vi "OrientationStateMachine.vi"(8 "Rubik's Moves":T1, 11 "Initial Orientation":T2) -> (3 "Final Orientation":T2)   [LabVIEW 2017]
uses:
  Controls/OrientationState.ctl
  Controls/RubikMoves.ctl
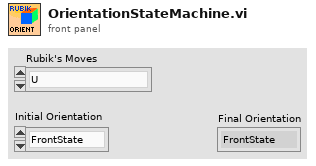
[diagram p1: front panel]
types:
  T1 = typedef "RubikMoves.ctl" = enum16{"U", "U'", "F", "F'", "D", "D'", "B", "B'", "L", "L'", "R", "R'"}
  T2 = typedef "OrientationState.ctl" = enum16{"FrontState", "UpState", "BackState", "DownState"}
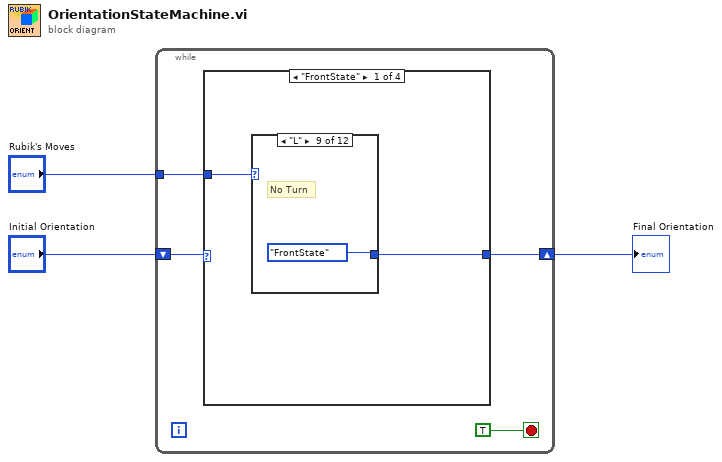
[diagram p0: block diagram]
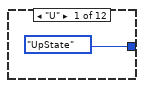
[diagram p2: hidden frame]
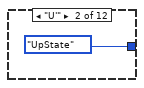
[diagram p3: hidden frame]
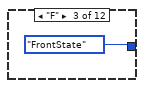
[diagram p4: hidden frame]
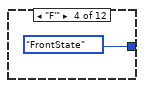
[diagram p5: hidden frame]
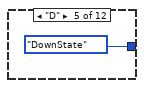
[diagram p6: hidden frame]
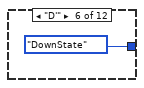
[diagram p7: hidden frame]
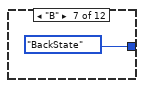
[diagram p8: hidden frame]
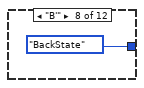
[diagram p9: hidden frame]
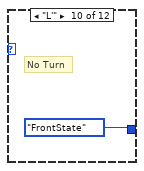
[diagram p10: hidden frame]
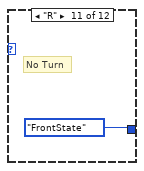
[diagram p11: hidden frame]
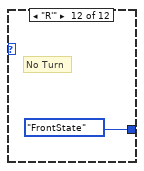
[diagram p12: hidden frame]
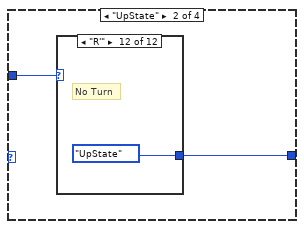
[diagram p13: hidden frame]
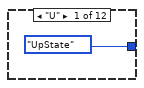
[diagram p14: hidden frame]
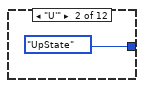
[diagram p15: hidden frame]
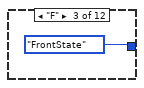
[diagram p16: hidden frame]
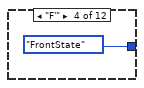
[diagram p17: hidden frame]
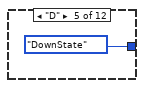
[diagram p18: hidden frame]
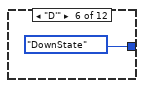
[diagram p19: hidden frame]
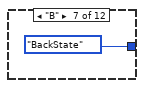
[diagram p20: hidden frame]
diagram:
  n1 = while {
    tunnel: "Rubik's Moves" -> [w7]
    shift-right: [w4] -> w2
    shift-left: "Initial Orientation" -> [w5]
    stop <- TRUE stop-if-true
    n2 = case shown="\"FrontState\"" w5 {
      tunnel: w7 -> [w9 w23 w37 w50]
      tunnel: [w8 w22 w36 w51] -> w4
      frame "FrontState" {
        n3 = case shown="\"L\"" w9 {
          tunnel: [OrientationState."UpState" ("Initial Orientation") OrientationState."UpState" ("Initial Orientation") OrientationState."FrontState" ("Initial Orientation") OrientationState."FrontState" ("Initial Orientation") OrientationState."DownState" ("Initial Orientation") OrientationState."DownState" ("Initial Orientation") OrientationState."BackState" ("Initial Orientation") OrientationState."BackState" ("Initial Orientation") OrientationState."FrontState" ("Initial Orientation") OrientationState."FrontState" ("Initial Orientation") OrientationState."FrontState" ("Initial Orientation") OrientationState."FrontState" ("Initial Orientation")] -> w8
          frame "U" {
          }
          frame "U'" {
          }
          frame "F" {
          }
          frame "F'" {
          }
          frame "D" {
          }
          frame "D'" {
          }
          frame "B" {
          }
          frame "B'" {
          }
          frame "L" {
            # "No Turn"
          }
          frame "L'" {
            # "No Turn"
          }
          frame "R" {
            # "No Turn"
          }
          frame "R'" {
            # "No Turn"
          }
        }
      }
      frame "UpState" {
        n4 = case shown="\"R'\"" w23 {
          tunnel: [OrientationState."UpState" ("Initial Orientation") OrientationState."UpState" ("Initial Orientation") OrientationState."FrontState" ("Initial Orientation") OrientationState."FrontState" ("Initial Orientation") OrientationState."DownState" ("Initial Orientation") OrientationState."DownState" ("Initial Orientation") OrientationState."BackState" ("Initial Orientation") OrientationState."BackState" ("Initial Orientation") OrientationState."UpState" ("Initial Orientation") OrientationState."UpState" ("Initial Orientation") OrientationState."UpState" ("Initial Orientation") OrientationState."UpState" ("Initial Orientation")] -> w22
          frame "U" {
          }
          frame "U'" {
          }
          frame "F" {
          }
          frame "F'" {
          }
          frame "D" {
          }
          frame "D'" {
          }
          frame "B" {
          }
          frame "B'" {
          }
          frame "L" {
            # "No Turn"
          }
          frame "L'" {
            # "No Turn"
          }
          frame "R" {
            # "No Turn"
          }
          frame "R'" {
            # "No Turn"
          }
        }
      }
      frame "BackState" {
        n5 = case shown="\"L\"" w37 {
          tunnel: [OrientationState."UpState" ("Initial Orientation") OrientationState."UpState" ("Initial Orientation") OrientationState."FrontState" ("Initial Orientation") OrientationState."FrontState" ("Initial Orientation") OrientationState."DownState" ("Initial Orientation") OrientationState."DownState" ("Initial Orientation") OrientationState."BackState" ("Initial Orientation") OrientationState."BackState" ("Initial Orientation") OrientationState."BackState" ("Initial Orientation") OrientationState."BackState" ("Initial Orientation") OrientationState."BackState" ("Initial Orientation") OrientationState."BackState" ("Initial Orientation")] -> w36
          frame "U" {
          }
          frame "U'" {
          }
          frame "F" {
          }
          frame "F'" {
          }
          frame "D" {
          }
          frame "D'" {
          }
          frame "B" {
          }
          frame "B'" {
          }
          frame "L" {
            # "No Turn"
          }
          frame "L'" {
            # "No Turn"
          }
          frame "R" {
            # "No Turn"
          }
          frame "R'" {
            # "No Turn"
          }
        }
      }
      frame "DownState" {
        n6 = case shown="\"L\"" w50 {
          tunnel: [OrientationState."UpState" ("Initial Orientation") OrientationState."UpState" ("Initial Orientation") OrientationState."FrontState" ("Initial Orientation") OrientationState."FrontState" ("Initial Orientation") OrientationState."DownState" ("Initial Orientation") OrientationState."DownState" ("Initial Orientation") OrientationState."BackState" ("Initial Orientation") OrientationState."BackState" ("Initial Orientation") OrientationState."DownState" ("Initial Orientation") OrientationState."DownState" ("Initial Orientation") OrientationState."DownState" ("Initial Orientation") OrientationState."DownState" ("Initial Orientation")] -> w51
          frame "U" {
          }
          frame "U'" {
          }
          frame "F" {
          }
          frame "F'" {
          }
          frame "D" {
          }
          frame "D'" {
          }
          frame "B" {
          }
          frame "B'" {
          }
          frame "L" {
            # "No Turn"
          }
          frame "L'" {
            # "No Turn"
          }
          frame "R" {
            # "No Turn"
          }
          frame "R'" {
            # "No Turn"
          }
        }
      }
    }
  }
  "Final Orientation" <- w2
